vi "Onda triangular con Arreglos de datos.vi"() -> ()   [LabVIEW 2014]
uses:
  <vilib>/LabVIEW Interface for Arduino/Type Defs/Pin Mode.ctl
  <vilib>/LabVIEW Interface for Arduino/LabVIEW Interface for Arduino.lvlib
panel:
  in  "VISA resource name":refnum<visa-resource-name>
  out "Waveform Chart":dynamicdata(graph)
  in  "Slide":i32(slide) scale=0.0..100.0
  # "Preset"
  # "Signal Visualization"
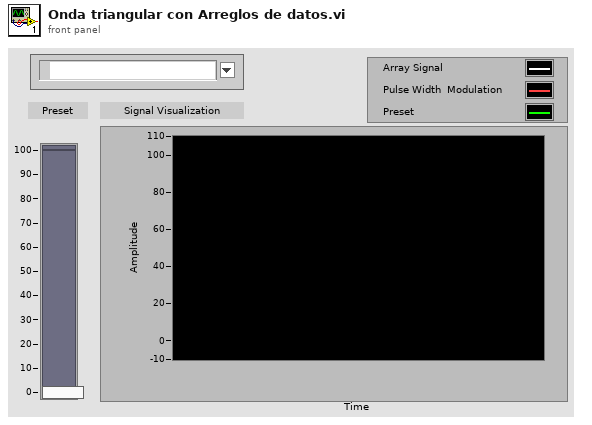
[diagram p1: front panel]
types:
  T1 = typedef "LabVIEW Interface for Arduino.lvlib/Pin Mode.ctl" = enum8{"Input", "Output"}
  T2 = typedef "LabVIEW Interface for Arduino.lvlib/Arduino Resource.ctl" = cluster{"VISA resource":refnum<visa-resource-name>, "Board Type":T3, "Connection Type":enum8{"USB / Serial"}, "Bytes Per Packet (15)":u8}
  T3 = typedef "LabVIEW Interface for Arduino.lvlib/Board Type.ctl" = enum16{"Uno", "Dimuelanove w/Atmega 328", "Mega 2560"}
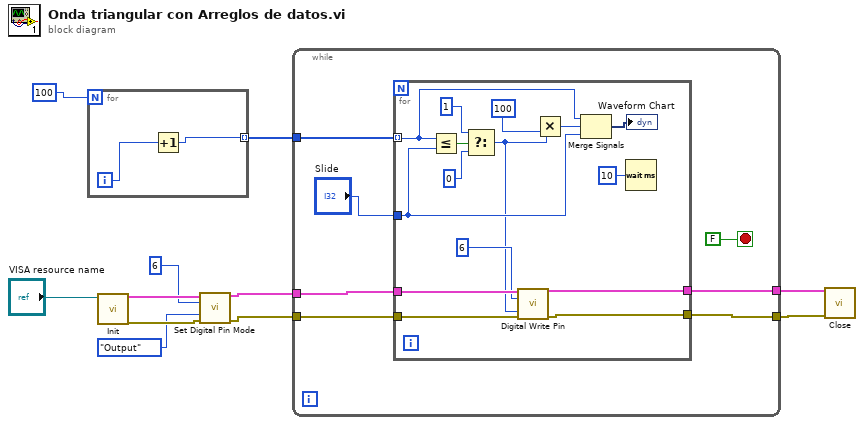
[diagram p0: block diagram]
diagram:
  n1 = for {
    N: 100 -> [_]
    tunnel: [w12] -> w10 mode=indexing
    i -> [w13]
    n2 = Increment(x=w13) -> (x+1=w12:i32)
  }
  n3 = call <vilib>:"Init.vi"("VISA resource"="VISA resource name") -> ("Arduino Resource"=w8:T2, "error out"=w7:errorcluster)  [unwired: 17 in]
  n4 = call <vilib>:"Set Digital Pin Mode.vi"("Arduino Resource"=w8, "Digital I/O Pin"=u8 6, "Pin Mode (Input)"=Pin_Mode."Output", "error in"=w7) -> ("Arduino Resource"=w6:T2, "error out"=w5:errorcluster)  [unwired: 10 in]
  n5 = while {
    tunnel: w10 -> [w20]
    tunnel: w6 -> [w17]
    tunnel: w5 -> [w16]
    tunnel: [w15] -> w4
    tunnel: [w14] -> w3
    stop <- FALSE stop-if-true
    n6 = for {
      tunnel: w20 -> [w28] mode=indexing
      tunnel: "Slide" -> [w30]
      tunnel: w17 -> [w26]
      tunnel: w16 -> [w25]
      tunnel: [w24] -> w15
      tunnel: [w23] -> w14
      n7 = Less Or Equal?(x=w28, y=w30) -> (x <= y?=w34:bool)
      n8 = Select(t=u8 1, s=w34, f=u8 0) -> (s? t:f=w21:u8)
      n9 = call <vilib>:"Digital Write Pin.vi"("Arduino Resource"=w26, "Digital I/O Pin (0)"=u8 6, "Value (0)"=w21, "error in"=w25) -> ("Arduino Resource"=w23:T2, "error out"=w24:errorcluster)  [unwired: 10 in]
      n10 = Multiply(x=w21, y=u8 100) -> (x*y=w29:u8)
      n11 = Merge Signals(w28, w29, w30) -> (→"Waveform Chart":dynamicdata)
      n12 = Wait (ms)(milliseconds to wait=u32 10) -> ()  [unwired: 1 out]
    }
  }
  n13 = call <vilib>:"Close.vi"("Arduino Resource"=w3, "error in"=w4) -> ()  [unwired: 13 in, 1 out]
